vi "senor caña.vi"() -> ()   [LabVIEW 2017]
panel:
  out "sensor caña":bool
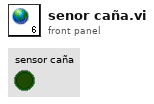
[diagram p1: front panel]
diagram:
